vi "SSL Detection Balls Delete Invalids.vi"(5 "Now":timestamp, 7 "Life Time":dbl=1.0, 11 "Balls In":T1[](array[typedef])) -> (3 "Balls Out":T1[](array[typedef]))   [LabVIEW 2017]
uses:
  SSL Detection Ball.ctl
  <vilib>/Analysis/Matrix/Datatypes/RealMatrix.ctl
  <vilib>/Analysis/Matrix/NI_Matrix.lvlib
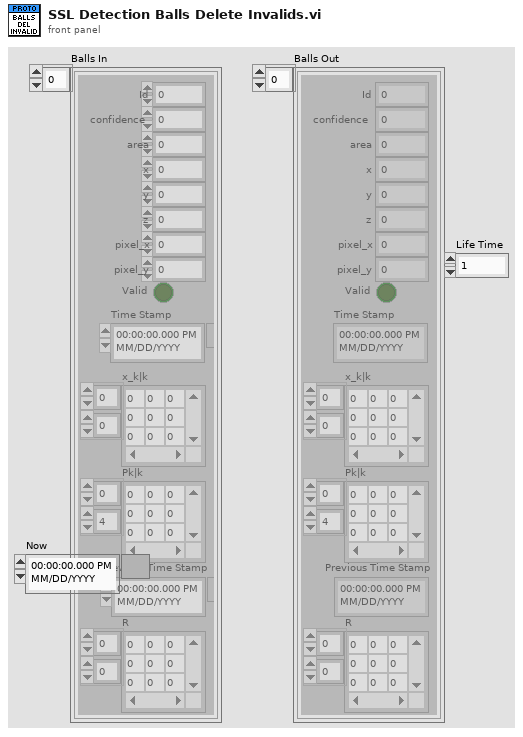
[diagram p1: front panel]
types:
  T1 = typedef "SSL Detection Ball.ctl" = cluster{"x":sgl, "area":u32, "confidence":sgl, "y":sgl, "z":sgl, "pixel_x":sgl, "pixel_y":sgl, "Valid":bool, "Time Stamp":timestamp, "x_k|k":T2, "Pk|k":T2, "Id":u32, "Previous Time Stamp":timestamp, "R":T2}
  T2 = typedef "NI_Matrix.lvlib/RealMatrix.ctl" = dbl[][]
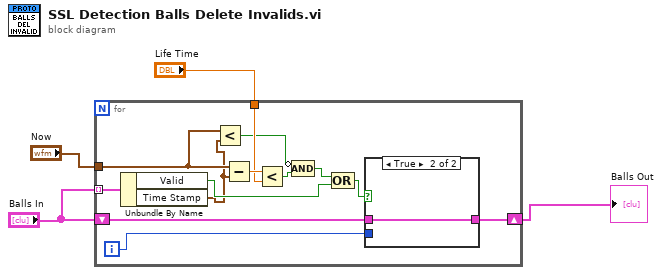
[diagram p0: block diagram]
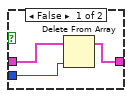
[diagram p2: hidden frame]
diagram:
  n1 = for {
    tunnel: "Balls In" -> [w17] mode=indexing
    shift-right: [w14] -> w4
    shift-left: "Balls In" -> [w16]
    tunnel: "Now" -> [w9]
    tunnel: "Life Time" -> [w12]
    i -> [w15]
    n2 = Unbundle By Name(w17) -> ("Valid"=w11:bool, "Time Stamp"=w8:timestamp)
    n3 = Less?(x=w9, y=w8) -> (x < y?=w6:bool)
    n4 = Subtract(x=w9, y=w8) -> (x-y=w13:dbl)
    n5 = Less?(x=w13, y=w12) -> (x < y?=w7:bool)
    n6 = Compound Arithmetic op=AND(invert w6, w7) -> (w5:bool)
    n7 = Compound Arithmetic op=OR(w5, w11) -> (w10:bool)
    n8 = case shown="True" w10 {
      tunnel: w16 -> [w20 w21]
      tunnel: w15 -> [w19 _]
      tunnel: [w18 w21] -> w14
      frame False {
        n9 = Delete From Array(array=w20, index=w19) -> (array with subset deleted=w18:T1[])  [unwired: 1 in, 1 out]
      }
      frame True {
      }
    }
  }
  "Balls Out" <- w4
